vi "E8257C_ampl.vi"(1 "error in":errorcluster, 2 "Amplitude dBm":dbl=10.0 min=0.00025 max=40.0 step=0.001 format="%.9f", 3 "GPIB address":string="19") -> (0 "error out":errorcluster)   [LabVIEW 2009]
panel:
  # "This VI controls Agilent E8257C PSG Analog Signal Generator \n  Set Frequency in CW mode"
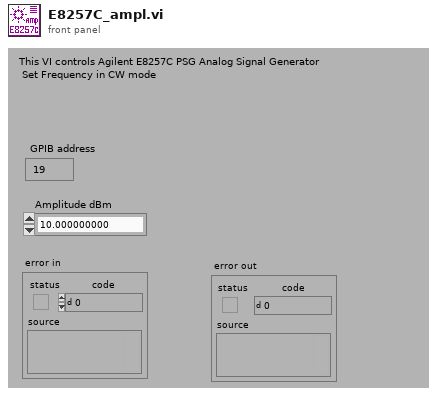
[diagram p1: front panel]
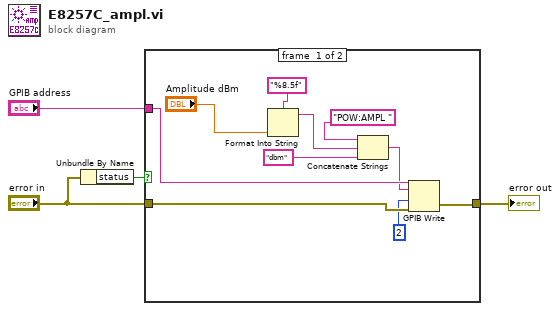
[diagram p0: block diagram]
diagram:
  n1 = Unbundle By Name("error in") -> ("status"=w4:bool)
  n2 = case shown="False" w4 {
    tunnel: "error in" -> [w10 w15]
    tunnel: [w11 w15] -> w2
    tunnel: "GPIB address" -> [w9 _]
    frame #0 {
      n3 = Format Into String(format string="%8.5f", "Amplitude dBm") -> (resulting string=w13:string)  [unwired: 2 in, 1 out]
      n4 = Concatenate Strings("POW:AMPL ", w13, "dbm") -> (w8:string)
      n5 = GPIB Write(0:w9, 1:w8, 2:i16 2 ("mode (0)"), 3:w10) -> (6:w11:errorcluster)  [unwired: 1 in, 1 out]
    }
    frame #1 {
    }
  }
  "error out" <- w2
